vi "Read Record Data.vi"(8 "Error In (no error)":errorcluster, 11 "Expenses Tracker Transaction In":refnum<class "Expenses Tracker Transaction.lvclass">) -> (0 "Error Out":errorcluster, 2 "Record":variant, 3 "Expenses Tracker Transaction Out":refnum<class "Expenses Tracker Transaction.lvclass">)   [LabVIEW 2023, in "Expenses Tracker Transaction.lvclass"]
uses:
  Expenses Tracker Transaction.lvclass
  Expenses Tracker Transaction.lvclass/Expenses Tracker Transaction.ctl
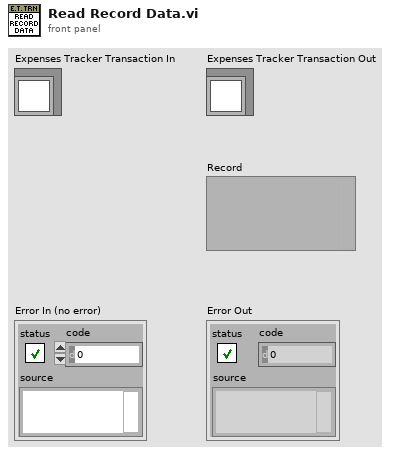
[diagram p1: front panel]
types:
  T1 = typedef "Expenses Tracker Record.lvclass/Transaction.ctl" = cluster{"ID":u32, "Name":string, "Is_income":bool, "Value":dbl, "Amount":dbl, "Total":dbl, "Date_of_entry":timestamp, "Date":timestamp, "Last_update":timestamp, "Category":u32, "Subcategory":u32, "Cycle":u32, "Description":string}
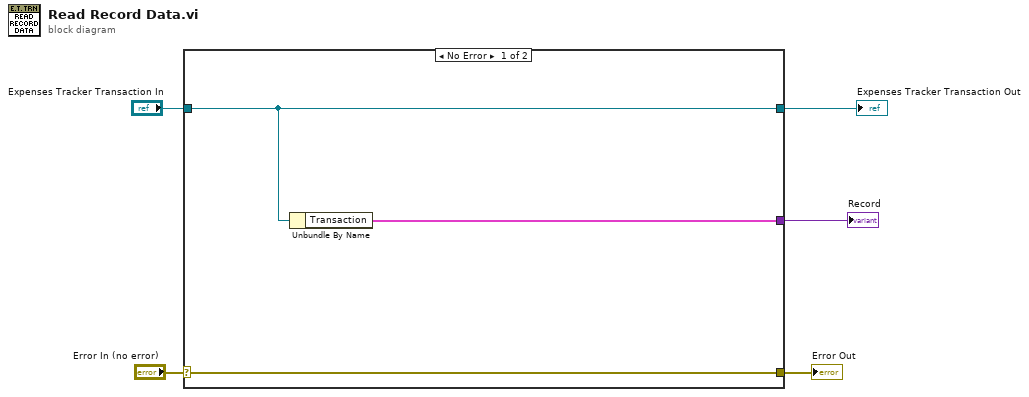
[diagram p0: block diagram]
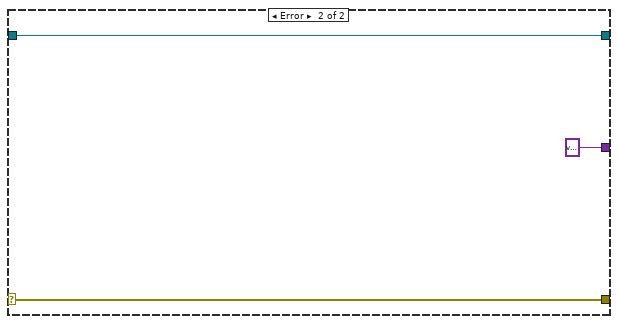
[diagram p2: hidden frame]
diagram:
  n1 = case shown="No Error" "Error In (no error)" {
    selector: "Error In (no error)" -> [w8 w11]
    tunnel: [w8 w11] -> w2
    tunnel: [w7 w10] -> w5
    tunnel: "Expenses Tracker Transaction In" -> [w7 w10]
    tunnel: [w6 variant] -> w1
    frame No Error {
      n2 = Unbundle By Name(w7) -> ("Transaction"=w6:T1)
    }
    frame Error {
    }
  }
  "Error Out" <- w2
  "Expenses Tracker Transaction Out" <- w5
  "Record" <- w1
